vi "Find Devices.vi"(0 "DeviceCount":i32, 1 "error in (no error)":errorcluster) -> (2 "DeviceCount out":i32, 3 "function return":i32, 4 "error out":errorcluster)   [LabVIEW 2014, in "ThorZStepper.lvlib"]
doc: "long FindDevices(long &DeviceCount);"
uses:
  ThorZStepper.lvlib
  ThorZStepper.dll
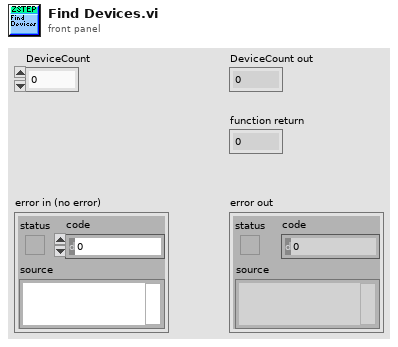
[diagram p1: front panel]
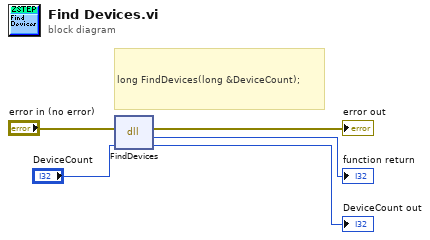
[diagram p0: block diagram]
diagram:
  # "long FindDevices(long &DeviceCount);"
  n1 = dll-call lib="C:/TIS_CalebVS2012/TIS_Development/Hardware/SDKs/MFC1_SDK/LabVIEW/inc/ThorZStepper.*" fn="FindDevices"(error in="error in (no error)", "DeviceCount"="DeviceCount") -> (error out=→"error out":errorcluster, "return type"=→"function return":i32, "DeviceCount"=→"DeviceCount out":i32)  [unwired: 2 in, 1 out]
